vi "S2C_LoadMenu.vi"(8 "Error In":errorcluster, 9 "Position":T1, 10 "MenuRef":refnum<k9>, 11 "CtlRef":refnum<vi>) -> (0 "Error Out":errorcluster, 3 "Discard?":bool)   [LabVIEW 2015]
doc: "Loads the menu associated with the selected build script cell."
uses:
  <vilib>/Utility/miscctls.llb/LVRowAndColumnTypeDef.ctl
  Globals/S2C_GlobalMenus.vi
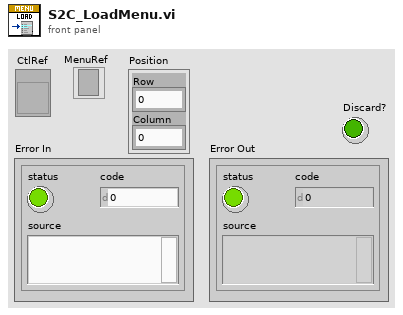
[diagram p1: front panel]
types:
  T1 = typedef "LVRowAndColumnTypeDef.ctl" = cluster{"Row":i32, "Column":i32}
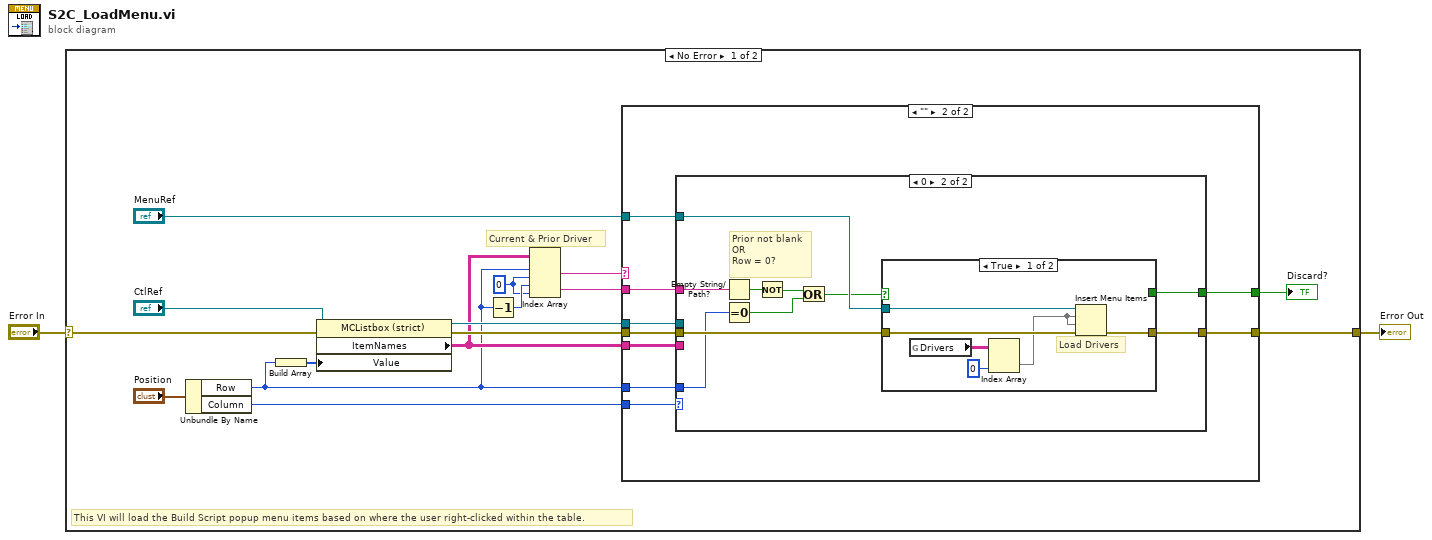
[diagram p0: block diagram]
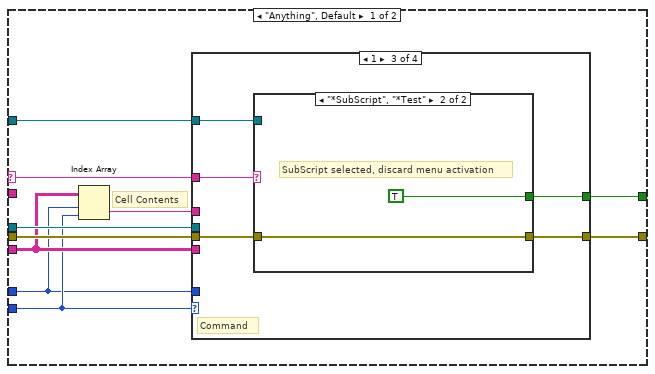
[diagram p2: hidden frame]
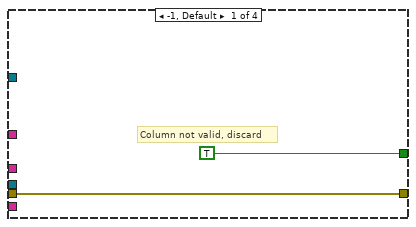
[diagram p3: hidden frame]
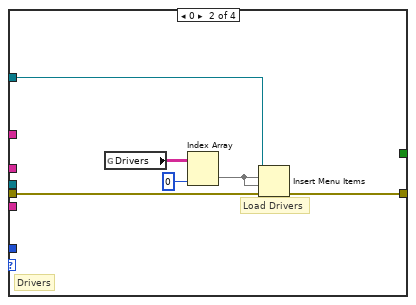
[diagram p4: hidden frame]
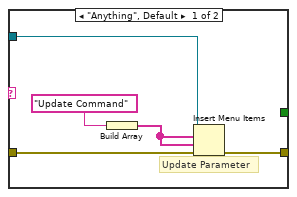
[diagram p5: hidden frame]
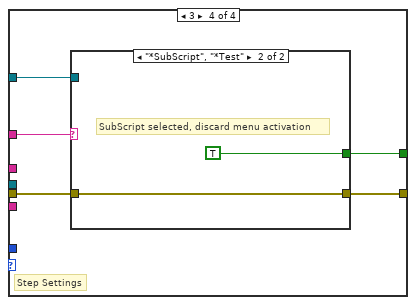
[diagram p6: hidden frame]
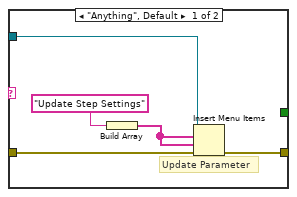
[diagram p7: hidden frame]
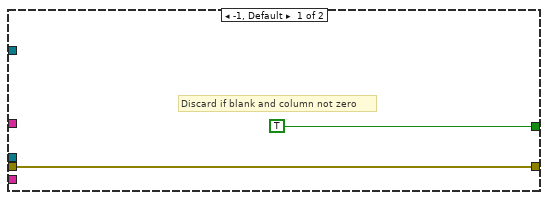
[diagram p8: hidden frame]
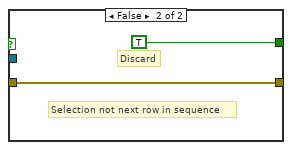
[diagram p9: hidden frame]
diagram:
  n1 = case shown="No Error" "Error In" {
    selector: "Error In" -> [w18 w90]
    tunnel: [w12 w90] -> w1
    frame No Error {
      w6 = 0 ("disabled index (col)")
      # "This VI will load the Build Script popup menu items based on where the user right-clicked within the table."
      # "Current & Prior Driver"
      n2 = Unbundle By Name("Position") -> ("Row"=w4:i32, "Column"=w17:i32)
      n3 = Build Array(w4) -> (w3:i32[])
      n4 = property on="Property Node" class="MCListbox (strict)"(reference="CtlRef", error in=w18, "Value"=w3) -> (reference out=w11:refnum<vi>, error out=w16:errorcluster, "ItemNames"=w9:string[][])
      n5 = Decrement(x=w4) -> (x-1=w7:i32)
      n6 = Index Array(array=w9, index (row) #1=w4, index (col) #1=w6, index (row) #2=w7, index (col) #2=w6) -> (element #1=w8:string, element #2=w5:string)
      n7 = case shown="\"\"" w8 {
        selector: w8 -> [w23 _]
        tunnel: w17 -> [w21 w69]
        tunnel: w16 -> [w28 w68]
        tunnel: "MenuRef" -> [w27 w67]
        tunnel: [w26 w66] -> w12
        tunnel: w11 -> [w25 w65]
        tunnel: [w24 w64] -> w10
        tunnel: w9 -> [w22 w63]
        tunnel: w4 -> [w20 w62]
        tunnel: w5 -> [_ w61]
        frame "Anything", Default {
          # "Cell Contents"
          n8 = Index Array(array=w22, index (row)=w20, index (col)=w21) -> (element=w19:string)
          n9 = case shown="1" w21 {
            tunnel: w28 -> [w30 w36 w39 w51]
            tunnel: w20 -> [_ _ _ _]
            tunnel: w27 -> [_ w35 w40 w52]
            tunnel: [w30 w34 w41 w53] -> w26
            tunnel: w22 -> [_ _ _ _]
            tunnel: [TRUE _ w37 w49] -> w24
            tunnel: w25 -> [_ _ _ _]
            tunnel: w23 -> [_ _ w38 w50]
            tunnel: w19 -> [_ _ _ _]
            frame -1, Default {
              # "Column not valid, discard"
            }
            frame 0 {
              # "Drivers"
              # "Load Drivers"
              n10 = global read "S2C_GlobalMenus.vi" "Drivers"() -> (w33:string[][])
              n11 = Index Array(array=w33, index (col)=0 ("disabled index (col)")) -> (element=w31:string[])  [unwired: 1 in]
              n12 = Insert Menu Items(6:w36, 7:w31, 8:w31, 9:w35) -> (0:w34:errorcluster)  [unwired: 2 in, 2 out]
            }
            frame 1 {
              # "Command"
              n13 = case shown="\"*SubScript\", \"*Test\"" w38 {
                tunnel: [w46 w48] -> w41
                tunnel: w40 -> [w45 _]
                tunnel: w39 -> [w44 w48]
                tunnel: [_ TRUE] -> w37
                frame "Anything", Default {
                  # "Update Parameter"
                  n14 = Build Array("Update Command") -> (w42:string[])
                  n15 = Insert Menu Items(6:w44, 7:w42, 8:w42, 9:w45) -> (0:w46:errorcluster)  [unwired: 2 in, 2 out]
                }
                frame "*SubScript", "*Test" {
                  # "SubScript selected, discard menu activation"
                }
              }
            }
            frame 3 {
              # "Step Settings"
              n16 = case shown="\"*SubScript\", \"*Test\"" w50 {
                tunnel: [w58 w60] -> w53
                tunnel: w52 -> [w57 _]
                tunnel: w51 -> [w56 w60]
                tunnel: [_ TRUE] -> w49
                frame "Anything", Default {
                  # "Update Parameter"
                  n17 = Build Array("Update Step Settings") -> (w54:string[])
                  n18 = Insert Menu Items(6:w56, 7:w54, 8:w54, 9:w57) -> (0:w58:errorcluster)  [unwired: 2 in, 2 out]
                }
                frame "*SubScript", "*Test" {
                  # "SubScript selected, discard menu activation"
                }
              }
            }
          }
        }
        frame "" {
          n19 = case shown="0" w69 {
            tunnel: w68 -> [w71 w81]
            tunnel: w62 -> [_ w74]
            tunnel: w67 -> [_ w79]
            tunnel: [w71 w80] -> w66
            tunnel: w63 -> [_ _]
            tunnel: [TRUE w78] -> w64
            tunnel: w65 -> [_ _]
            tunnel: w61 -> [_ w77]
            frame -1, Default {
              # "Discard if blank and column not zero"
            }
            frame 0 {
              # "Prior not blank\nOR\nRow = 0?"
              n20 = Empty String/Path?(string/path=w77) -> (empty?=w76:bool)
              n21 = Equal To 0?(x=w74) -> (x = 0?=w73:bool)
              n22 = Not(x=w76) -> (.not. x?=w75:bool)
              n23 = Or(x=w75, y=w73) -> (x .or. y?=w72:bool)
              n24 = case shown="True" w72 {
                tunnel: w81 -> [w87 w89]
                tunnel: [w86 w89] -> w80
                tunnel: w79 -> [w83 _]
                tunnel: [_ TRUE] -> w78
                frame True {
                  # "Load Drivers"
                  n25 = global read "S2C_GlobalMenus.vi" "Drivers"() -> (w85:string[][])
                  n26 = Index Array(array=w85, index (col)=0 ("disabled index (col)")) -> (element=w82:string[])  [unwired: 1 in]
                  n27 = Insert Menu Items(6:w87, 7:w82, 8:w82, 9:w83) -> (0:w86:errorcluster)  [unwired: 2 in, 2 out]
                }
                frame False {
                  # "Selection not next row in sequence"
                  # "Discard"
                }
              }
            }
          }
        }
      }
      "Discard?" <- w10
    }
    frame Error {
    }
  }
  "Error Out" <- w1
